vi "CalculateEQEandJsc.vi"(6 "Skip cell?":bool, 7 "Cell details cluster":T1={"Cell Position"=16, "Cell Label"="", "Pixel to measure"=0, "Area (cm^2)"=0.126, "Variable"="", "Variable value"="", "Scan settings in queue"=0, "Light or dark"="", "Measurement Type"=""} {"Pixel to measure" items=["All", "1", "2", "3", "4", "5", "6", "7", "8"]}, 8 "Max WL":string, 9 "Min WL":string, 10 "Ref meas file path":path, 11 "Pixel meas file path":path) -> (1 "Mismatch factor":dbl, 2 "Jsc at 1 sun (mA/cm^2)":dbl, 3 "EQE file path":path)   [LabVIEW 2016]
uses:
  <vilib>/Analysis/8numeric.llb/1D Numeric Integration.vi
  <vilib>/Utility/file.llb/Read From Spreadsheet File (DBL).vi
  <vilib>/Utility/file.llb/Write To Spreadsheet File (DBL).vi
  <vilib>/gmath/NI_Gmath.lvlib
  <vilib>/Analysis/NI_AALPro.lvlib
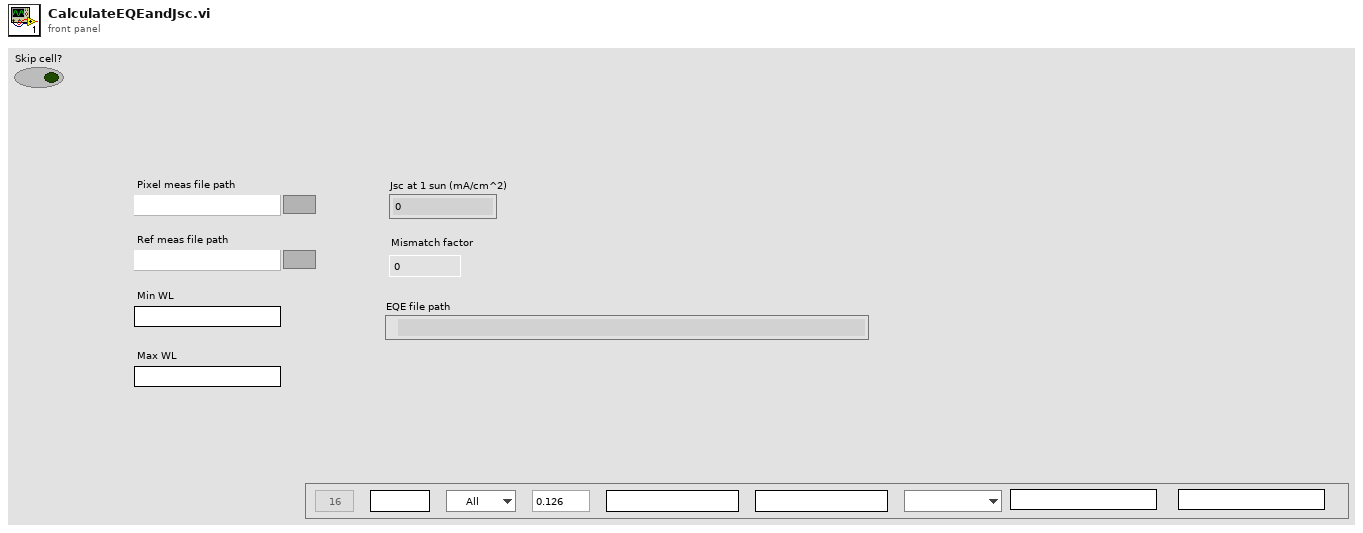
[diagram p1: front panel]
types:
  T1 = cluster{"Cell Position":i32, "Cell Label":string, "Pixel to measure":u16, "Area (cm^2)":dbl, "Variable":string, "Variable value":string, "Scan settings in queue":u16, "Light or dark":string, "Measurement Type":string}
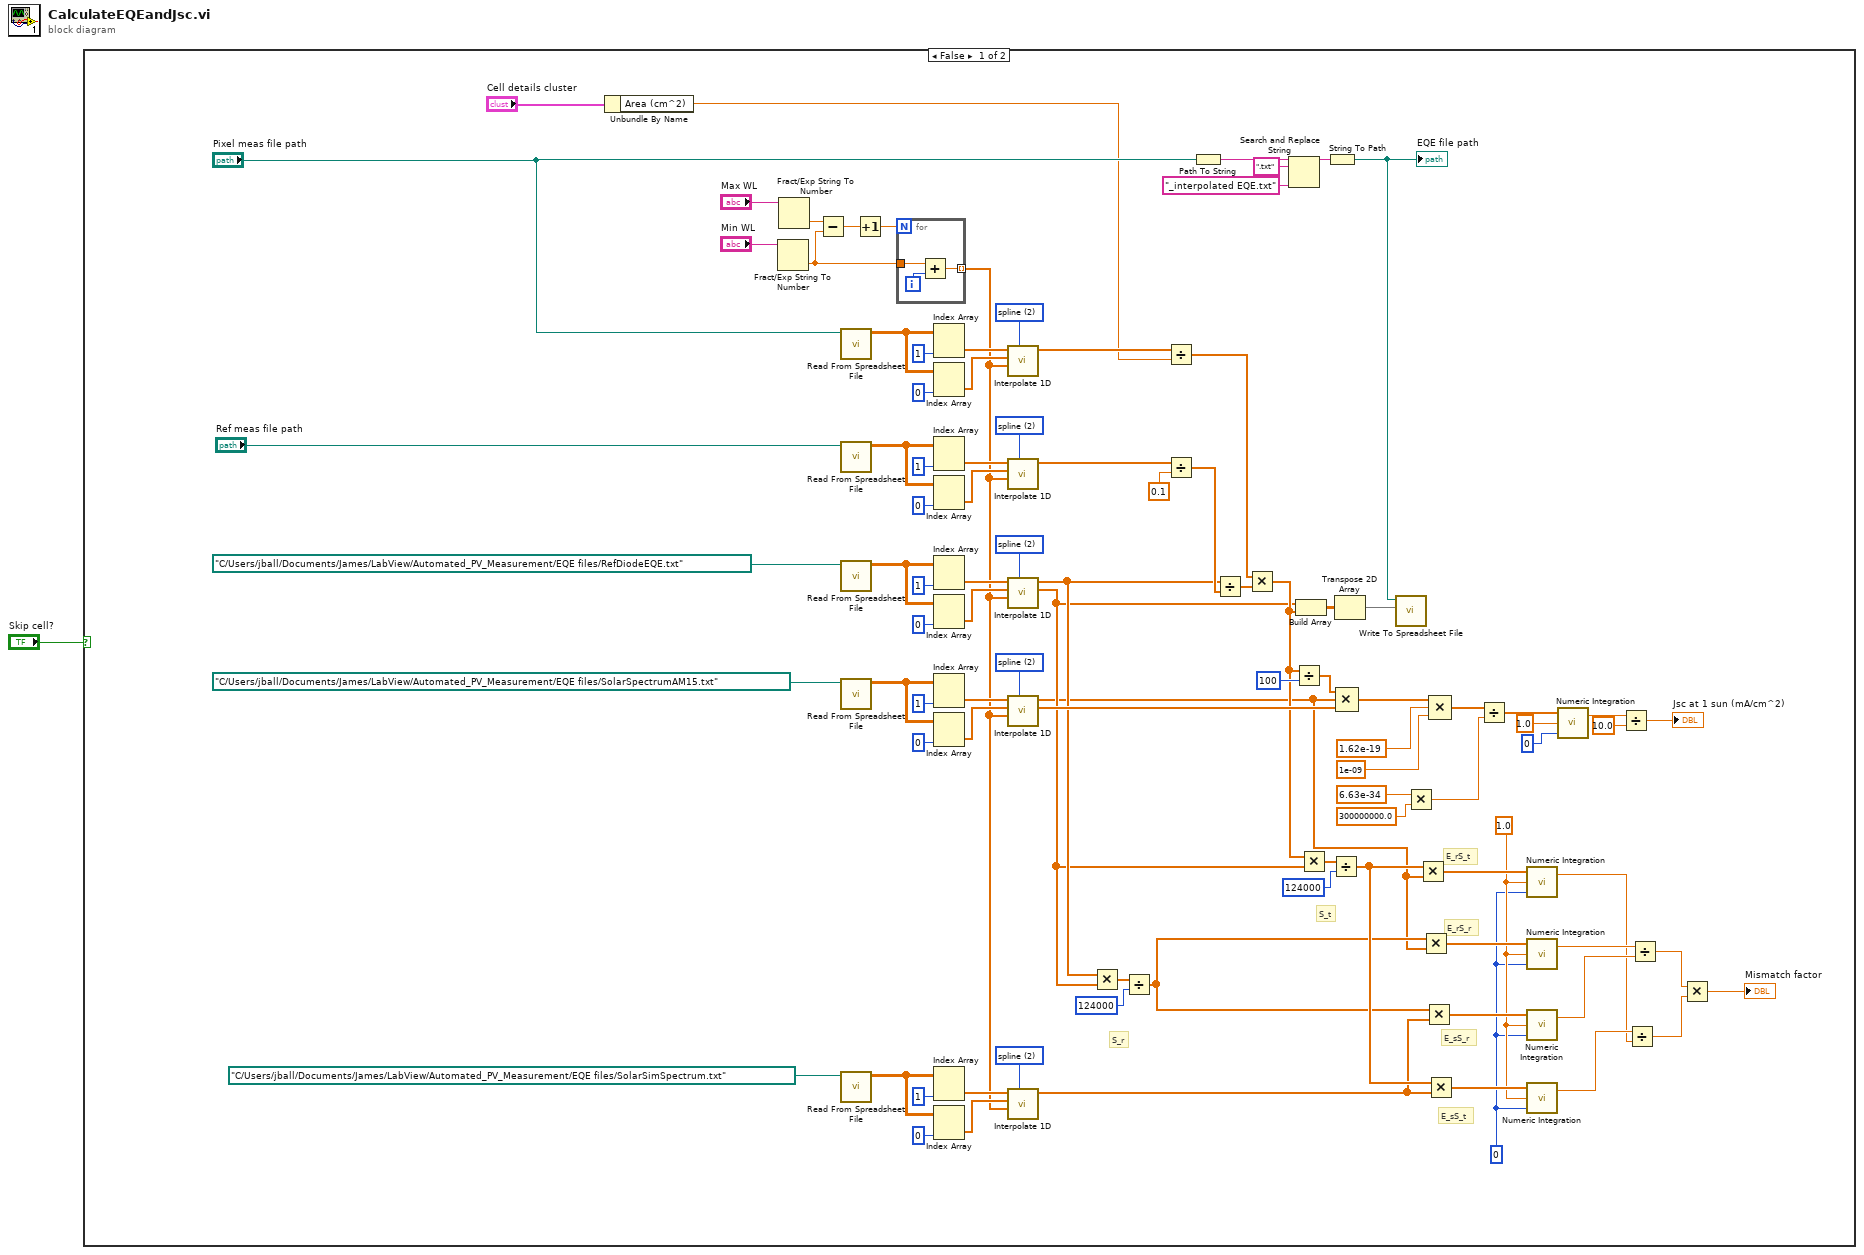
[diagram p0: block diagram]
diagram:
  n1 = case shown="False" "Skip cell?" {
    frame False {
      w11 = 0
      w12 = 1.0 ("dt")
      w33 = 2 items=["nearest", "linear", "spline", "cubic Hermite", "Lagrange"] ("method")
      w66 = 2 items=["nearest", "linear", "spline", "cubic Hermite", "Lagrange"] ("method")
      w80 = 2 items=["nearest", "linear", "spline", "cubic Hermite", "Lagrange"] ("method")
      w86 = 2 items=["nearest", "linear", "spline", "cubic Hermite", "Lagrange"] ("method")
      w91 = 2 items=["nearest", "linear", "spline", "cubic Hermite", "Lagrange"] ("method")
      # "E_sS_r"
      # "E_rS_r"
      # "E_sS_t"
      # "E_rS_t"
      # "S_t"
      # "S_r"
      n2 = Unbundle By Name("Cell details cluster") -> ("Area (cm^2)"=w2:dbl)
      n3 = Fract/Exp String To Number(string="Min WL") -> (number=w73:dbl)  [unwired: 3 in, 1 out]
      n4 = Fract/Exp String To Number(string="Max WL") -> (number=w75:dbl)  [unwired: 3 in, 1 out]
      n5 = Subtract(x=w75, y=w73) -> (x-y=w78:dbl)
      n6 = call-poly <vilib>:"Read From Spreadsheet File.vi"("file path (dialog if empty)"="Pixel meas file path") -> ("all rows"=w96:dbl[][])  [unwired: 6 in, 4 out]
      n7 = call-poly <vilib>:"Read From Spreadsheet File.vi"("file path (dialog if empty)"="Ref meas file path") -> ("all rows"=w85:dbl[][])  [unwired: 6 in, 4 out]
      n8 = call-poly <vilib>:"Read From Spreadsheet File.vi"("file path (dialog if empty)"=path "C:/Users/jball/Documents/James/LabView/Automated_PV_Measurement/EQE files/RefDiodeEQE.txt") -> ("all rows"=w65:dbl[][])  [unwired: 6 in, 4 out]
      n9 = call-poly <vilib>:"Read From Spreadsheet File.vi"("file path (dialog if empty)"=path "C:/Users/jball/Documents/James/LabView/Automated_PV_Measurement/EQE files/SolarSpectrumAM15.txt") -> ("all rows"=w79:dbl[][])  [unwired: 6 in, 4 out]
      n10 = call-poly <vilib>:"Read From Spreadsheet File.vi"("file path (dialog if empty)"=path "C:/Users/jball/Documents/James/LabView/Automated_PV_Measurement/EQE files/SolarSimSpectrum.txt") -> ("all rows"=w32:dbl[][])  [unwired: 6 in, 4 out]
      n11 = Increment(x=w78) -> (x+1=w77:dbl)
      n12 = for {
        N: w77 -> [_]
        tunnel: w73 -> [w100]
        tunnel: [w99] -> w31 mode=indexing
        i -> [w101]
        n13 = Add(x=w100, y=w101) -> (x+y=w99:dbl)
      }
      n14 = Index Array(array=w96, index (col)=1 ("disabled index (col)")) -> (element=w93:dbl[])  [unwired: 1 in]
      n15 = Index Array(array=w96, index (col)=0 ("disabled index (col)")) -> (element=w92:dbl[])  [unwired: 1 in]
      n16 = Index Array(array=w85, index (col)=1 ("disabled index (col)")) -> (element=w88:dbl[])  [unwired: 1 in]
      n17 = Index Array(array=w85, index (col)=0 ("disabled index (col)")) -> (element=w87:dbl[])  [unwired: 1 in]
      n18 = Index Array(array=w65, index (col)=1 ("disabled index (col)")) -> (element=w68:dbl[])  [unwired: 1 in]
      n19 = Index Array(array=w65, index (col)=0 ("disabled index (col)")) -> (element=w67:dbl[])  [unwired: 1 in]
      n20 = Index Array(array=w79, index (col)=1 ("disabled index (col)")) -> (element=w82:dbl[])  [unwired: 1 in]
      n21 = Index Array(array=w79, index (col)=0 ("disabled index (col)")) -> (element=w81:dbl[])  [unwired: 1 in]
      n22 = Index Array(array=w32, index (col)=1 ("disabled index (col)")) -> (element=w35:dbl[])  [unwired: 1 in]
      n23 = Index Array(array=w32, index (col)=0 ("disabled index (col)")) -> (element=w34:dbl[])  [unwired: 1 in]
      n24 = call <vilib>:"Interpolate 1D.vi"("method"=w91, "xi"=w31, "X"=w92, "Y"=w93) -> ("yi"=w72:dbl[])  [unwired: 5 in, 2 out]
      n25 = call <vilib>:"Interpolate 1D.vi"("method"=w86, "xi"=w31, "X"=w87, "Y"=w88) -> ("yi"=w64:dbl[])  [unwired: 5 in, 2 out]
      n26 = call <vilib>:"Interpolate 1D.vi"("method"=w66, "xi"=w31, "X"=w67, "Y"=w68) -> ("xi used"=w21:dbl[], "yi"=w27:dbl[])  [unwired: 5 in, 1 out]
      n27 = call <vilib>:"Interpolate 1D.vi"("method"=w80, "xi"=w31, "X"=w81, "Y"=w82) -> ("xi used"=w49:dbl[], "yi"=w18:dbl[])  [unwired: 5 in, 1 out]
      n28 = call <vilib>:"Interpolate 1D.vi"("method"=w33, "xi"=w31, "X"=w34, "Y"=w35) -> ("yi"=w17:dbl[])  [unwired: 5 in, 2 out]
      n29 = Multiply(x=w27, y=w21) -> (x*y=w25:dbl[])
      n30 = Divide(x=w25, y=124000 ("Numeric")) -> (x/y=w19:dbl[])
      n31 = Divide(x=w72, y=w2) -> (x/y=w60:dbl[])
      n32 = Divide(x=w64, y=0.1) -> (x/y=w62:dbl[])
      n33 = Path To String(path="Pixel meas file path") -> (string=w58:string)
      n34 = Divide(x=w27, y=w62) -> (x/y=w61:dbl[])
      n35 = Multiply(x=w60, y=w61) -> (x*y=w22:dbl[])
      n36 = Search and Replace String(input string=w58, search string=".txt", replace string="_interpolated EQE.txt" ("replace string (\"\")")) -> (result string=w59:string)  [unwired: 5 in, 3 out]
      n37 = Divide(x=w22, y=100) -> (x/y=w50:dbl[])
      n38 = Build Array(w21, w22) -> (w53:dbl[][])
      n39 = Multiply(x=w22, y=w21) -> (x*y=w23:dbl[])
      n40 = String To Path(string=w59) -> (path=w54:path)
      "EQE file path" <- w54
      n41 = Divide(x=w23, y=124000 ("Numeric")) -> (x/y=w20:dbl[])
      n42 = Transpose 2D Array(2D array=w53) -> (transposed array=w52:dbl[][])
      n43 = Compound Arithmetic op=MULTIPLY(w50, w18, w49) -> (w48:dbl[])
      n44 = call-poly <vilib>:"Write To Spreadsheet File.vi"("2D data"=w52, "file path (dialog if empty)"=w54) -> ()  [unwired: 6 in, 1 out]
      n45 = Multiply(x=6.63e-34, y=300000000.0) -> (x*y=w42:dbl)
      n46 = Multiply(x=w20, y=w18) -> (x*y=w16:dbl[])
      n47 = Multiply(x=w19, y=w18) -> (x*y=w15:dbl[])
      n48 = Multiply(x=w19, y=w17) -> (x*y=w14:dbl[])
      n49 = Multiply(x=w20, y=w17) -> (x*y=w13:dbl[])
      n50 = Compound Arithmetic op=MULTIPLY(w48, 1.62e-19, 1e-09) -> (w43:dbl[])
      n51 = Divide(x=w43, y=w42) -> (x/y=w41:dbl[])
      n52 = call-poly <vilib>:"Numeric Integration.vi"("integration method"=w11, "dt"=w12, "Input Array"=w16) -> ("result"=w6:dbl)  [unwired: 1 out]
      n53 = call-poly <vilib>:"Numeric Integration.vi"("integration method"=w11, "dt"=w12, "Input Array"=w15) -> ("result"=w9:dbl)  [unwired: 1 out]
      n54 = call-poly <vilib>:"Numeric Integration.vi"("integration method"=w11, "dt"=w12, "Input Array"=w14) -> ("result"=w8:dbl)  [unwired: 1 out]
      n55 = call-poly <vilib>:"Numeric Integration.vi"("integration method"=w11, "dt"=w12, "Input Array"=w13) -> ("result"=w7:dbl)  [unwired: 1 out]
      n56 = call-poly <vilib>:"Numeric Integration.vi"("integration method"=0, "dt"=1.0, "Input Array"=w41) -> ("result"=w30:dbl)  [unwired: 1 out]
      n57 = Divide(x=w30, y=10.0) -> (x/y=→"Jsc at 1 sun (mA/cm^2)":dbl)
      n58 = Divide(x=w7, y=w6) -> (x/y=w4:dbl)
      n59 = Divide(x=w9, y=w8) -> (x/y=w5:dbl)
      n60 = Multiply(x=w5, y=w4) -> (x*y=→"Mismatch factor":dbl)
    }
    frame True {
    }
  }
